vi "溶解氧电极校准.vi"() -> ()   [LabVIEW 2016, in "斯坦道多参数.lvlib"]
uses:
  <vilib>/Utility/miscctls.llb/LVPointTypeDef.ctl
  <vilib>/Analysis/NI_AALBase.lvlib
panel:
  out "第二点校准值":dbl
  out "第一点校准值":dbl
  out "最小值":sgl format="%#.2f"
  out "最大值":sgl format="%#.2f"
  in  "校准模式":enum16{"两点校准", "单点校准"}(ring)=enum."单点校准"
  in  "校准停止":bool
  in  "校准启动":bool
  out "波形图表":sgl(graph) caption="历史曲线"
  out "变异系数":dbl format="%#.6f"
  out "standard deviation":dbl caption="标准差" format="%#.2f"
  out "mean":dbl caption="均值" format="%#.2f"
  out "测量读值":dbl
  out "偏移值补偿":dbl
  out "饱和度值":dbl
  out "提示":string
  out "气压补偿值":dbl
  out "盐度补偿值":dbl
  out "电极斜率":dbl
  out "电极零点":dbl
  # "溶解氧电极设定"
  # "%"
  # "%"
  # "%"
  # "mg/L"
  # "ppt"
  # "hPa"
  # "mg/L"
  # "请选择校准模式:"
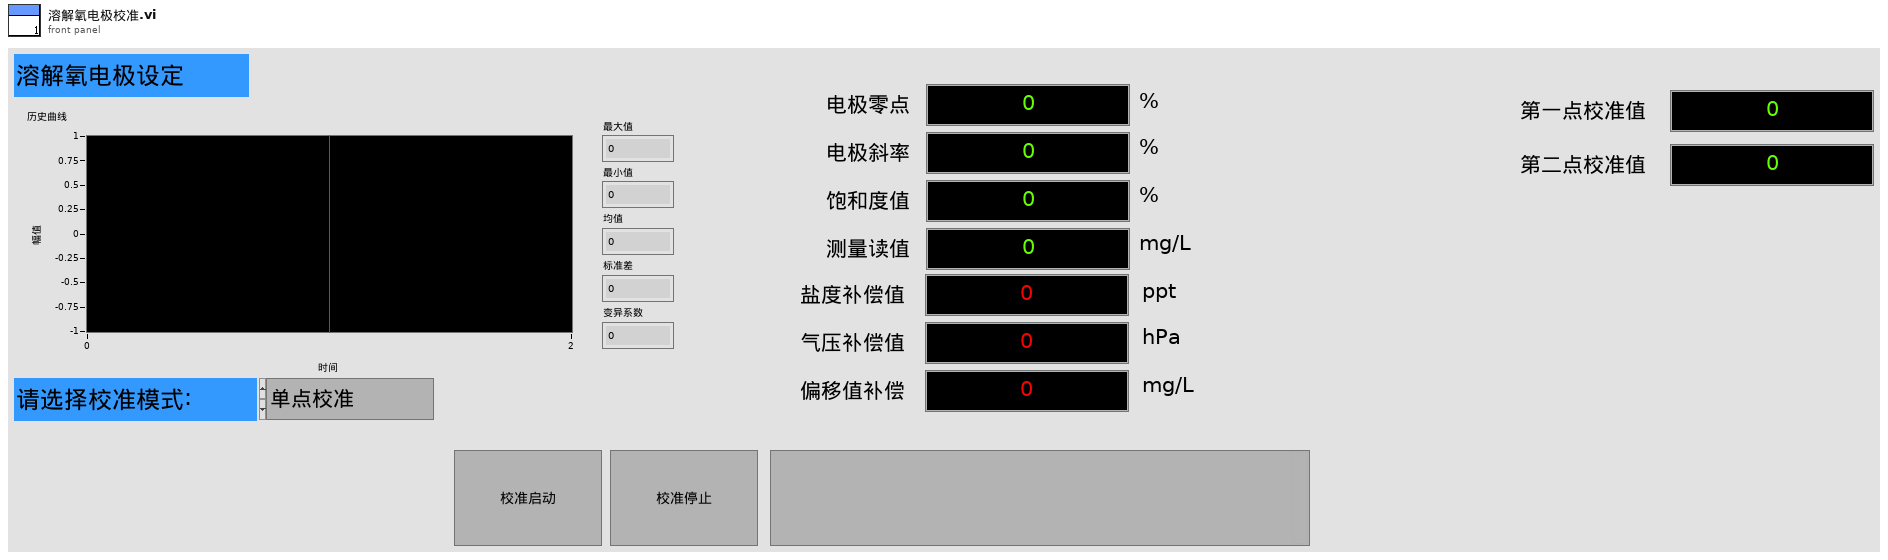
[diagram p1: front panel]
types:
  T1 = typedef "斯坦道多参数.lvlib/校准步骤.ctl" = enum16{"待机", "放置第一点标液", "第一点校准启动", "第一点校准写入", "第一点校准失败", "放置第二点标液", "第二点校准启动", "第二点校准写入", "第二点校准失败", "放置第三点标液", "第三点校准启动", "第三点校准写入", "第三点校准失败", "校准结果写入", "校准结束"}
  T2 = typedef "LVPointTypeDef.ctl" = cluster{"Horizontal":i16, "Vertical":i16}
  T3 = cluster{"电极状态标志":u16, "电极型号标志":u16, "溶解氧测量值":sgl, "温度测量值":sgl, "溶解氧饱和度值":sgl, "盐度补偿值":sgl, "大气压补偿值":sgl, "溶解氧偏移修正值":sgl, "温度偏移修正值":sgl, "手动温度补偿值":sgl, "溶解氧电极零点":sgl, "溶解氧电极斜率":sgl, "第1点标准值记录":sgl, "第1点信号值记录":sgl, "第1点温度值记录":sgl, "第2点标准值记录":sgl, "第2点信号值记录":sgl, "第2点温度值记录":sgl, "命令滤波设定":u16, "温度模式":enum16{"ATC", "MTC"}, "生产批次":u16, "电极序号":u16, "串口地址":u16, "串口波特率":enum16{"9600", "19200", "115200"}, "串口校验位":enum16{"NONE", "ODD", "EVEN"}, "串口停止位":enum16{"1bit", "2bit"}, "第一点标准值":sgl, "第二点标准值":sgl}
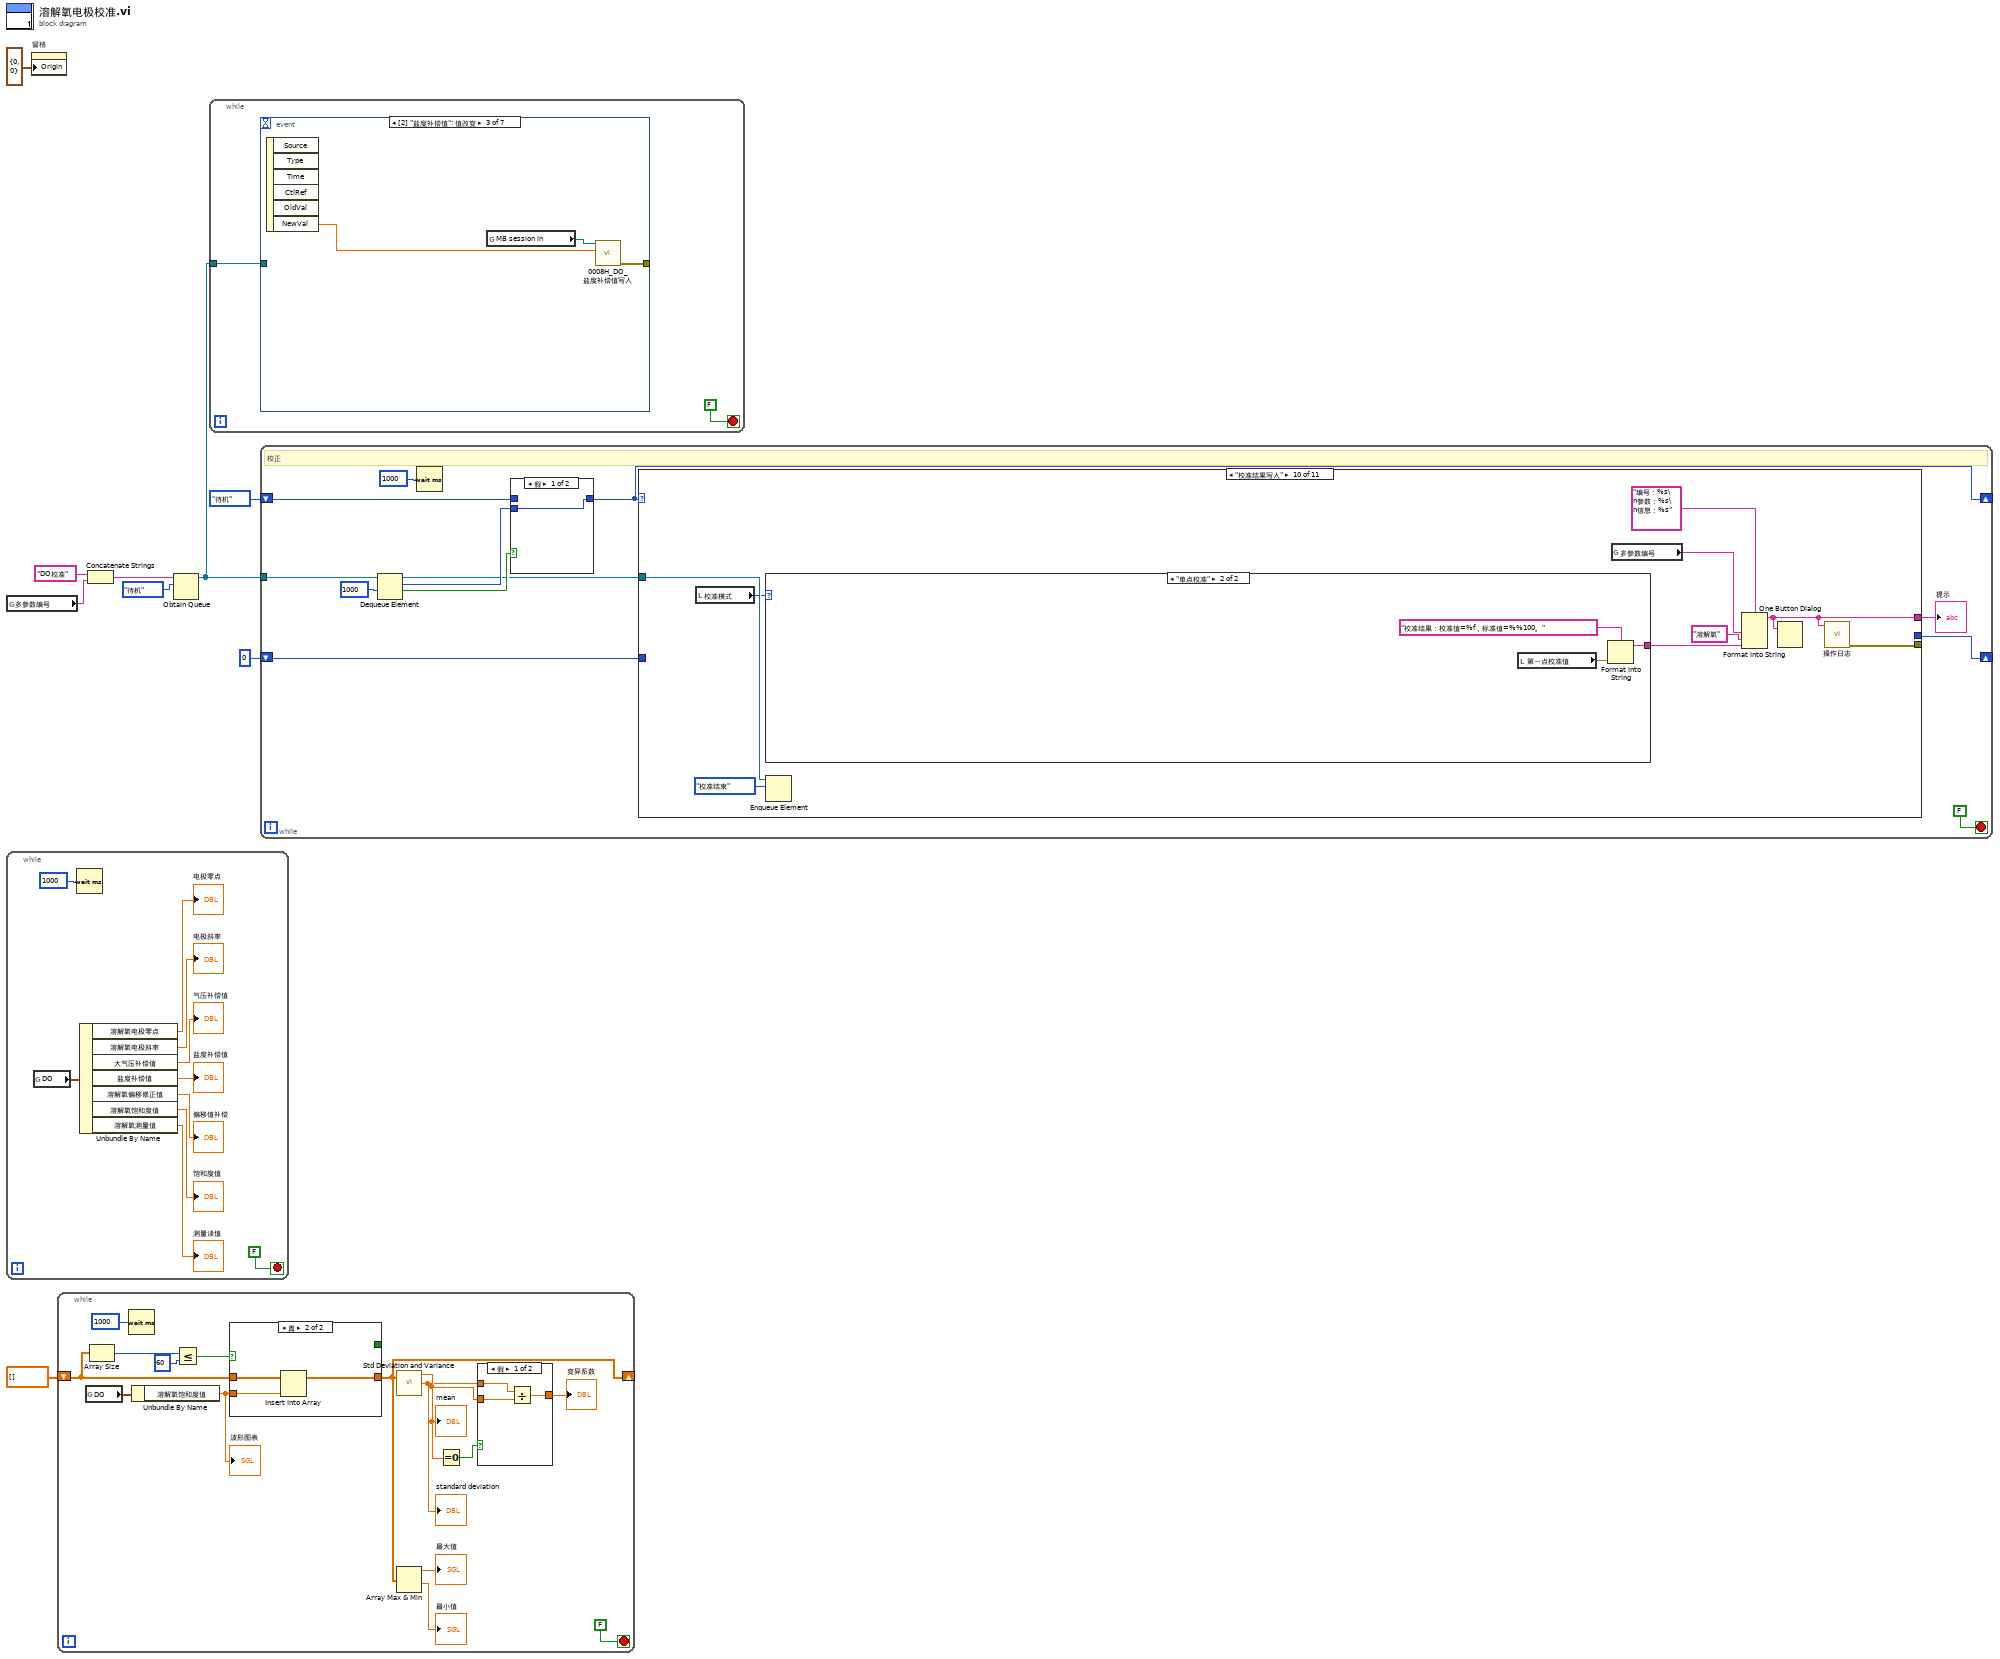
[diagram p0: block diagram]
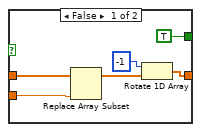
[diagram p3: hidden frame]
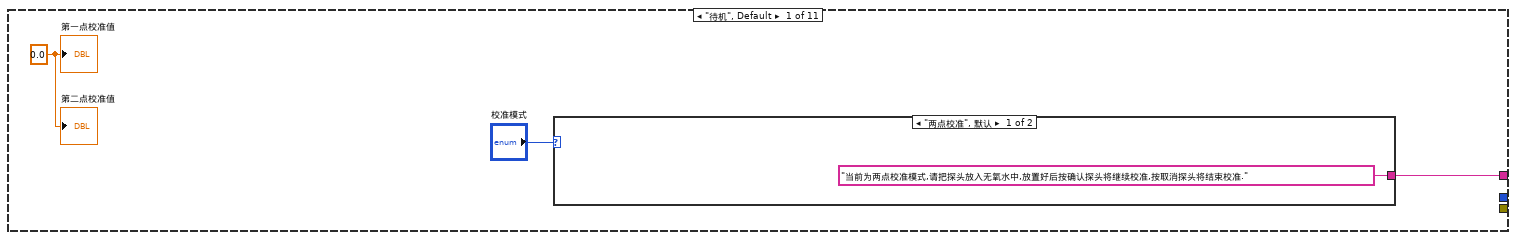
[diagram p5: hidden frame]
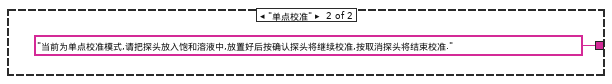
[diagram p6: hidden frame]
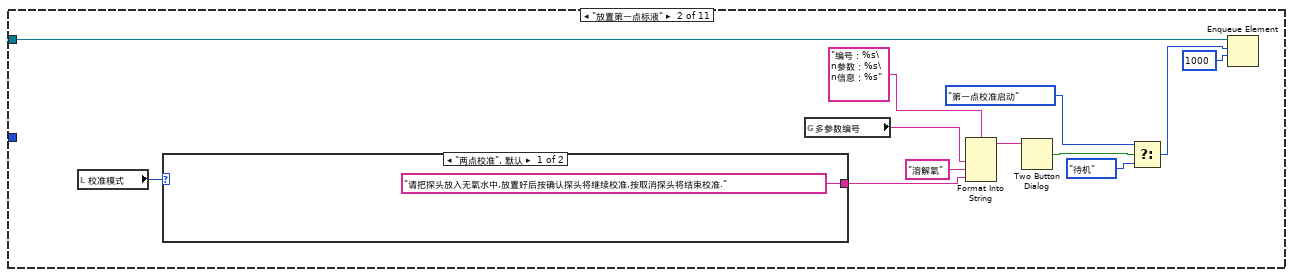
[diagram p7: hidden frame]
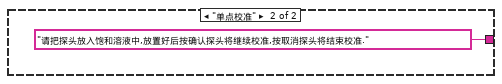
[diagram p8: hidden frame]
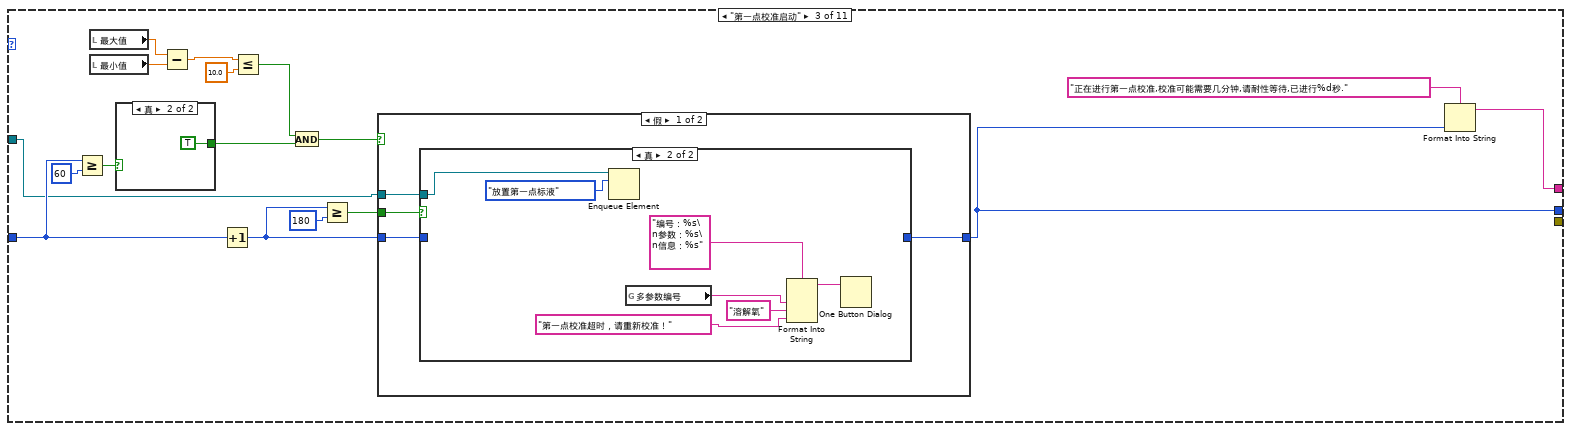
[diagram p9: hidden frame]
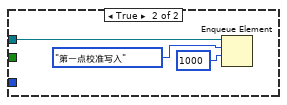
[diagram p11: hidden frame]
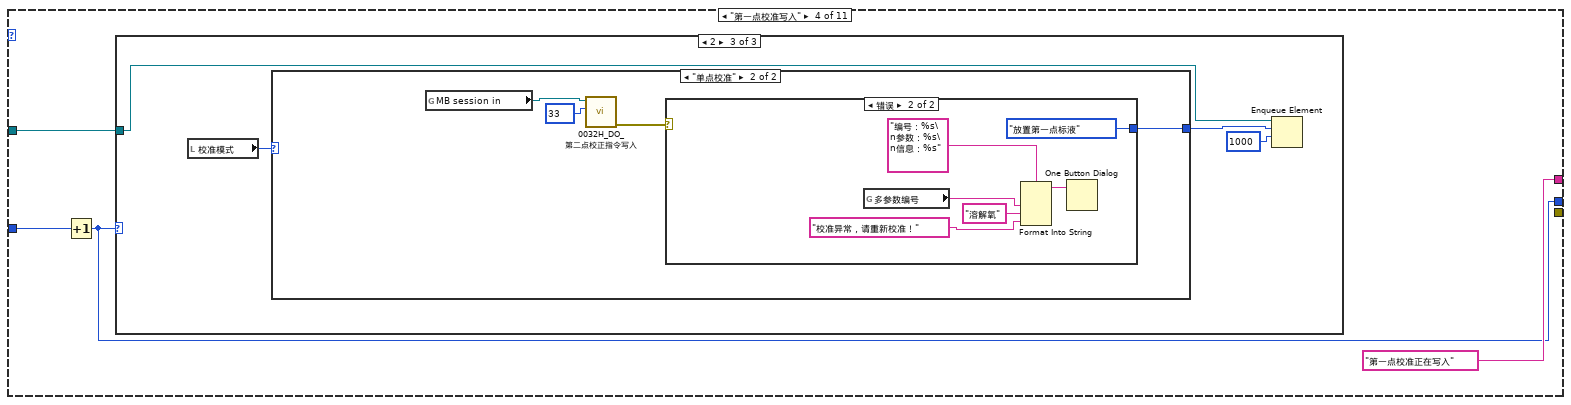
[diagram p13: hidden frame]
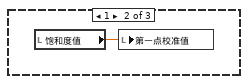
[diagram p15: hidden frame]
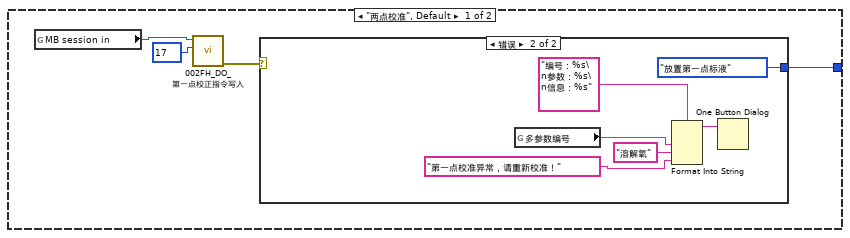
[diagram p16: hidden frame]
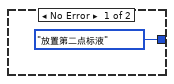
[diagram p17: hidden frame]
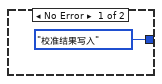
[diagram p18: hidden frame]
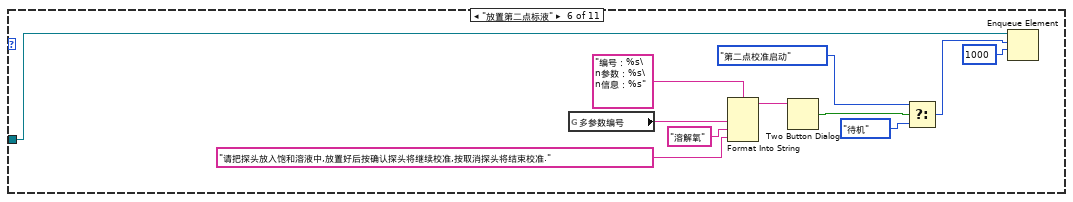
[diagram p20: hidden frame]
diagram:
  n1 = global read "多参数全局变量.vi" "多参数编号"() -> (w1:string)
  n2 = while {
    stop <- FALSE stop-if-true
    n3 = global read "国弘过程全局变量.vi" "DO"() -> (w17:T3)
    n4 = Wait (ms)(milliseconds to wait=u32 1000 ("等待时间（毫秒）")) -> ()  [unwired: 1 out]
    n5 = Unbundle By Name(w17) -> ("溶解氧电极零点"=→"电极零点":sgl, "溶解氧电极斜率"=→"电极斜率":sgl, "大气压补偿值"=→"气压补偿值":sgl, "盐度补偿值"=→"盐度补偿值":sgl, "溶解氧偏移修正值"=→"偏移值补偿":sgl, "溶解氧饱和度值"=→"饱和度值":sgl, "溶解氧测量值"=→"测量读值":sgl)
  }
  n6 = property on="窗格" class="Pane"("Origin"=T2 {"Horizontal"=0, "Vertical"=0} ("原点")) -> ()  [unwired: 2 in, 2 out]
  n7 = while {
    shift-right: [w23] -> _
    shift-left: sgl[] [] -> [w30]
    stop <- FALSE stop-if-true
    n8 = global read "国弘过程全局变量.vi" "DO"() -> (w26:T3)
    n9 = Array Size(array=w30) -> (size(s)=w32:i32)
    n10 = Wait (ms)(milliseconds to wait=u32 1000 ("等待时间（毫秒）")) -> ()  [unwired: 1 out]
    n11 = Unbundle By Name(w26) -> ("溶解氧饱和度值"=w20:sgl)
    "波形图表" <- w20
    n12 = Less Or Equal?(x=w32, y=60) -> (x <= y?=w31:bool)
    n13 = case shown="真" w31 {
      tunnel: w30 -> [w43 w46]
      tunnel: w20 -> [w41 w45]
      tunnel: [w39 w44] -> w23
      tunnel: [TRUE _] -> _
      frame False {
        n14 = Replace Array Subset(array=w43, new element=w41) -> (w42:sgl[])  [unwired: 1 in]
        n15 = Rotate 1D Array(1:w42, 2:-1 ("n")) -> (0:w39:sgl[])
      }
      frame True {
        n16 = Insert Into Array(array=w46, new element=w45) -> (w44:sgl[])  [unwired: 1 in]
      }
    }
    n17 = call <vilib>:"Std Deviation and Variance.vi"("X"=w23) -> ("mean"=w25:dbl, "standard deviation"=w24:dbl)  [unwired: 1 in, 1 out]
    "mean" <- w25
    "standard deviation" <- w24
    n18 = Array Max & Min(array=w23) -> (max value=→"最大值":sgl, min value=→"最小值":sgl)  [unwired: 2 out]
    n19 = Equal To 0?(x=w25) -> (x = 0?=w29:bool)
    n20 = case shown="假" w29 {
      tunnel: w24 -> [w37 _]
      tunnel: [w36 _] -> w28
      tunnel: w25 -> [w35 _]
      frame False {
        n21 = Divide(x=w37, y=w35) -> (x/y=w36:dbl)
      }
      frame True {
      }
    }
    "变异系数" <- w28
  }
  n22 = Concatenate Strings("DO校准" ("名称（未命名）"), w1) -> (w2:string)
  n23 = Obtain Queue(name (unnamed)=w2, element data type=校准步骤."待机" ("枚举")) -> (queue out=w3:refnum<queue>)  [unwired: 3 in, 2 out]
  n24 = while {
    tunnel: w3 -> [w47]
    stop <- FALSE stop-if-true
    n25 = event shown="[2] \"盐度补偿值\": 值改变" {
      selector: _ -> [_ _ _ _ _ _ _]
      dyn-events: _ -> [_ _ _ _ _ _ _]
      timeout: _ -> [_ _ _ _ _ _ _]
      tunnel: [_ _ w54 w57 w60 _ _] -> _
      tunnel: w47 -> [_ _ _ _ _ w62 w64]
      event Timeout {
        n26 = event-data() -> ()  [unwired: 1 in, 3 out]
      }
      event "盐度补偿值", "气压补偿值", "偏移值补偿": Mouse Down {
        n27 = event-data() -> ("CtlRef"=w50:refnum<vi>)  [unwired: 1 in, 7 out]
        n28 = property class="DigNum (严格)"(reference=w50) -> (reference out=w49:refnum<vi>, "Value"=w51:dbl)  [unwired: 1 in, 1 out]
        n29 = call "数字键盘.vi"("OldNumber"=w51) -> ("NewNumber"=w52:dbl)  [unwired: 1 in]
        n30 = property class="DigNum (严格)"(reference=w49, "Val(Sgnl)"=w52) -> ()  [unwired: 1 in, 2 out]
      }
      event "盐度补偿值": Value Change {
        n31 = event-data() -> ("NewVal"=w55:dbl)  [unwired: 1 in, 5 out]
        n32 = global read "多参数全局变量.vi" "MB session in"() -> (w53:refnum<class "MB_Master.lvclass">)
        n33 = call "0008H_DO_盐度补偿值写入.vi"("数值"=w55, "MB session in"=w53) -> ("error out"=w54:errorcluster)  [unwired: 8 in, 1 out]
      }
      event "气压补偿值": Value Change {
        n34 = event-data() -> ("NewVal"=w58:dbl)  [unwired: 1 in, 5 out]
        n35 = global read "多参数全局变量.vi" "MB session in"() -> (w56:refnum<class "MB_Master.lvclass">)
        n36 = call "000AH_DO_大气压补偿值写入.vi"("数值"=w58, "MB session in"=w56) -> ("error out"=w57:errorcluster)  [unwired: 8 in, 1 out]
      }
      event "偏移值补偿": Value Change {
        n37 = event-data() -> ("NewVal"=w61:dbl)  [unwired: 1 in, 5 out]
        n38 = global read "多参数全局变量.vi" "MB session in"() -> (w59:refnum<class "MB_Master.lvclass">)
        n39 = call "000CH_DO_DO偏移修正值写入.vi"("数值"=w61, "MB session in"=w59) -> ("error out"=w60:errorcluster)  [unwired: 8 in, 1 out]
      }
      event "校准启动": Value Change {
        n40 = event-data() -> ()  [unwired: 1 in, 6 out]
        n41 = Enqueue Element(queue=w62, element=校准步骤."放置第一点标液" ("元素")) -> ()  [unwired: 2 in, 3 out]
      }
      event "校准停止": Value Change {
        n42 = event-data() -> ()  [unwired: 1 in, 6 out]
        n43 = Flush Queue(queue=w64) -> (queue out=w65:refnum<queue>)  [unwired: 1 in, 2 out]
        n44 = Enqueue Element(queue=w65, element=校准步骤."待机" ("元素"), timeout in ms (-1)=1000 ("超时毫秒(-1)")) -> ()  [unwired: 1 in, 3 out]
      }
    }
  }
  n45 = while "While循环" {
    shift-right: [w69] -> _
    shift-left: 校准步骤."待机" ("枚举") -> [w70]
    shift-right: [w76] -> _
    shift-left: 0 -> [w77]
    tunnel: w3 -> [w71]
    stop <- FALSE stop-if-true
    # "校正"
    n46 = Dequeue Element(queue=w71, timeout in ms (-1)=1000 ("超时毫秒(-1)")) -> (queue out=w68:refnum<queue>, element=w72:T1, timed out?=w73:bool)  [unwired: 1 in, 1 out]
    n47 = Wait (ms)(milliseconds to wait=u32 1000 ("等待时间（毫秒）")) -> ()  [unwired: 1 out]
    n48 = case shown="假" w73 {
      tunnel: w72 -> [w80 _]
      tunnel: [w80 w81] -> w69
      tunnel: w70 -> [_ w81]
      frame False {
      }
      frame True {
      }
    }
    n49 = case shown="\"校准结果写入\"" w69 {
      tunnel: [w84 _ w105 "第一点校准正在写入" ("提示") _ _ w177 "第二点校准正在写入" ("提示") _ w227 w255] -> w75
      tunnel: w77 -> [_ _ w109 w136 _ _ w179 w211 _ _ _]
      tunnel: [_ _ w108 w135 _ _ w178 w210 _ _ _] -> w76
      tunnel: w68 -> [_ w93 w107 w134 _ w170 w180 w209 _ w234 _]
      tunnel: [_ _ _ _ _ _ _ _ _ w232 _] -> _
      frame "待机", Default {
        w82 = 0.0 ("第一点校准值")
        n50 = case shown="\"两点校准\", 默认" "校准模式" {
          tunnel: ["当前为两点校准模式,请把探头放入无氧水中,放置好后按确认探头将继续校准,按取消探头将结束校准." ("消息") "当前为单点校准模式,请把探头放入饱和溶液中,放置好后按确认探头将继续校准,按取消探头将结束校准." ("消息")] -> w84
          frame "两点校准", Default {
          }
          frame "单点校准" {
          }
        }
        "第一点校准值" <- w82
        "第二点校准值" <- w82
      }
      frame "放置第一点标液" {
        n51 = local read "校准模式"() -> (w92:enum16{"两点校准", "单点校准"})
        n52 = case shown="\"两点校准\", 默认" w92 {
          tunnel: ["请把探头放入无氧水中,放置好后按确认探头将继续校准,按取消探头将结束校准." ("消息") "请把探头放入饱和溶液中,放置好后按确认探头将继续校准,按取消探头将结束校准." ("消息")] -> w87
          frame "两点校准", Default {
          }
          frame "单点校准" {
          }
        }
        n53 = global read "多参数全局变量.vi" "多参数编号"() -> (w90:string)
        n54 = Format Into String(format string="编号：%s\n参数：%s\n信息：%s" ("格式字符串"), w90, "溶解氧" ("输入 2"), w87) -> (resulting string=w88:string)  [unwired: 2 in, 1 out]
        n55 = Two Button Dialog(message=w88) -> (T button?=w97:bool)  [unwired: 2 in]
        n56 = Select(t=校准步骤."第一点校准启动" ("元素"), s=w97, f=校准步骤."待机" ("元素")) -> (s? t:f=w94:T1)
        n57 = Enqueue Element(queue=w93, element=w94, timeout in ms (-1)=1000 ("超时毫秒(-1)")) -> ()  [unwired: 1 in, 3 out]
      }
      frame "第一点校准启动" {
        n58 = Greater Or Equal?(x=w109, y=60) -> (x >= y?=w116:bool)
        n59 = local read "最大值"() -> (w113:sgl)
        n60 = local read "最小值"() -> (w112:sgl)
        n61 = case shown="真" w116 {
          tunnel: [_ TRUE] -> w104
          frame False {
          }
          frame True {
          }
        }
        n62 = Subtract(x=w113, y=w112) -> (x-y=w114:sgl)
        n63 = Increment(x=w109) -> (x+1=w106:i32)
        n64 = Less Or Equal?(x=w114, y=10.0) -> (x <= y?=w103:bool)
        n65 = And(x=w103, y=w104) -> (x .and. y?=w102:bool)
        n66 = Greater Or Equal?(x=w106, y=180) -> (x >= y?=w110:bool)
        n67 = case shown="假" w102 {
          tunnel: w107 -> [w120 w132]
          tunnel: w110 -> [w121 _]
          tunnel: w106 -> [w119 _]
          tunnel: [w118 _] -> w108
          frame False {
            n68 = case shown="真" w121 {
              tunnel: w120 -> [_ w129]
              tunnel: w119 -> [w122 _]
              tunnel: [w122 _] -> w118
              frame False {
              }
              frame True {
                n69 = Enqueue Element(queue=w129, element=校准步骤."放置第一点标液" ("元素")) -> ()  [unwired: 2 in, 3 out]
                n70 = global read "多参数全局变量.vi" "多参数编号"() -> (w126:string)
                n71 = Format Into String(format string="编号：%s\n参数：%s\n信息：%s" ("格式字符串"), w126, "溶解氧" ("输入 2"), "第一点校准超时，请重新校准！" ("error source (\" \")")) -> (resulting string=w124:string)  [unwired: 2 in, 1 out]
                n72 = One Button Dialog(message=w124) -> ()  [unwired: 1 in, 1 out]
              }
            }
          }
          frame True {
            n73 = Enqueue Element(queue=w132, element=校准步骤."第一点校准写入" ("元素"), timeout in ms (-1)=1000 ("超时毫秒(-1)")) -> ()  [unwired: 1 in, 3 out]
          }
        }
        n74 = Format Into String(format string="正在进行第一点校准,校准可能需要几分钟,请耐性等待,已进行%d秒." ("格式字符串"), w108) -> (resulting string=w105:string)  [unwired: 2 in, 1 out]
      }
      frame "第一点校准写入" {
        n75 = Increment(x=w136) -> (x+1=w135:i32)
        n76 = case shown="2" w135 {
          tunnel: w134 -> [_ _ w140]
          frame 0, Default {
          }
          frame 1 {
            n77 = local read "饱和度值"() -> (w138:dbl)
            n78 = local write "第一点校准值"(w138) -> ()
          }
          frame 2 {
            n79 = local read "校准模式"() -> (w142:enum16{"两点校准", "单点校准"})
            n80 = case shown="\"单点校准\"" w142 {
              tunnel: [w143 w154] -> w139
              frame "两点校准", Default {
                n81 = global read "多参数全局变量.vi" "MB session in"() -> (w144:refnum<class "MB_Master.lvclass">)
                n82 = call "002FH_DO_第一点校正指令写入.vi"("数值"=u16 17, "MB session in"=w144) -> ("error out"=w145:errorcluster)  [unwired: 8 in, 1 out]
                n83 = case shown="错误" w145 {
                  tunnel: [校准步骤."放置第二点标液" ("元素") 校准步骤."放置第一点标液" ("元素")] -> w143
                  frame No Error {
                  }
                  frame Error {
                    n84 = global read "多参数全局变量.vi" "多参数编号"() -> (w151:string)
                    n85 = Format Into String(format string="编号：%s\n参数：%s\n信息：%s" ("格式字符串"), w151, "溶解氧" ("输入 2"), "第一点校准异常，请重新校准！" ("error source (\" \")")) -> (resulting string=w149:string)  [unwired: 2 in, 1 out]
                    n86 = One Button Dialog(message=w149) -> ()  [unwired: 1 in, 1 out]
                  }
                }
              }
              frame "单点校准" {
                n87 = global read "多参数全局变量.vi" "MB session in"() -> (w156:refnum<class "MB_Master.lvclass">)
                n88 = call "0032H_DO_第二点校正指令写入.vi"("数值"=u16 33, "MB session in"=w156) -> ("error out"=w155:errorcluster)  [unwired: 8 in, 1 out]
                n89 = case shown="错误" w155 {
                  tunnel: [校准步骤."校准结果写入" ("元素") 校准步骤."放置第一点标液" ("元素")] -> w154
                  frame No Error {
                  }
                  frame Error {
                    n90 = global read "多参数全局变量.vi" "多参数编号"() -> (w162:string)
                    n91 = Format Into String(format string="编号：%s\n参数：%s\n信息：%s" ("格式字符串"), w162, "溶解氧" ("输入 2"), "校准异常，请重新校准！" ("error source (\" \")")) -> (resulting string=w161:string)  [unwired: 2 in, 1 out]
                    n92 = One Button Dialog(message=w161) -> ()  [unwired: 1 in, 1 out]
                  }
                }
              }
            }
            n93 = Enqueue Element(queue=w140, element=w139, timeout in ms (-1)=1000 ("超时毫秒(-1)")) -> ()  [unwired: 1 in, 3 out]
          }
        }
      }
      frame "第一点校准失败" {
      }
      frame "放置第二点标液" {
        n94 = global read "多参数全局变量.vi" "多参数编号"() -> (w168:string)
        n95 = Format Into String(format string="编号：%s\n参数：%s\n信息：%s" ("格式字符串"), w168, "溶解氧" ("输入 2"), "请把探头放入饱和溶液中,放置好后按确认探头将继续校准,按取消探头将结束校准." ("消息")) -> (resulting string=w165:string)  [unwired: 2 in, 1 out]
        n96 = Two Button Dialog(message=w165) -> (T button?=w174:bool)  [unwired: 2 in]
        n97 = Select(t=校准步骤."第二点校准启动" ("元素"), s=w174, f=校准步骤."待机" ("元素")) -> (s? t:f=w171:T1)
        n98 = Enqueue Element(queue=w170, element=w171, timeout in ms (-1)=1000 ("超时毫秒(-1)")) -> ()  [unwired: 1 in, 3 out]
      }
      frame "第二点校准启动" {
        n99 = Greater Or Equal?(x=w179, y=60) -> (x >= y?=w191:bool)
        n100 = local read "最大值"() -> (w188:sgl)
        n101 = local read "最小值"() -> (w187:sgl)
        n102 = case shown="真" w191 {
          tunnel: [_ TRUE] -> w184
          frame False {
          }
          frame True {
          }
        }
        n103 = Subtract(x=w188, y=w187) -> (x-y=w189:sgl)
        n104 = Increment(x=w179) -> (x+1=w185:i32)
        n105 = Less Or Equal?(x=w189, y=10.0) -> (x <= y?=w183:bool)
        n106 = And(x=w183, y=w184) -> (x .and. y?=w182:bool)
        n107 = Greater Or Equal?(x=w185, y=180) -> (x >= y?=w186:bool)
        n108 = case shown="假" w182 {
          tunnel: w180 -> [w195 w207]
          tunnel: w186 -> [w196 _]
          tunnel: w185 -> [w194 _]
          tunnel: [w193 _] -> w178
          frame False {
            n109 = case shown="真" w196 {
              tunnel: w195 -> [_ w204]
              tunnel: w194 -> [w197 _]
              tunnel: [w197 _] -> w193
              frame False {
              }
              frame True {
                n110 = Enqueue Element(queue=w204, element=校准步骤."放置第二点标液" ("元素")) -> ()  [unwired: 2 in, 3 out]
                n111 = global read "多参数全局变量.vi" "多参数编号"() -> (w201:string)
                n112 = Format Into String(format string="编号：%s\n参数：%s\n信息：%s" ("格式字符串"), w201, "溶解氧" ("输入 2"), "第二点校准超时，请重新校准！" ("error source (\" \")")) -> (resulting string=w199:string)  [unwired: 2 in, 1 out]
                n113 = One Button Dialog(message=w199) -> ()  [unwired: 1 in, 1 out]
              }
            }
          }
          frame True {
            n114 = Enqueue Element(queue=w207, element=校准步骤."第二点校准写入" ("元素"), timeout in ms (-1)=1000 ("超时毫秒(-1)")) -> ()  [unwired: 1 in, 3 out]
          }
        }
        n115 = Format Into String(format string="正在进行第二点校准,校准可能需要几分钟,请耐性等待,已进行%d秒." ("格式字符串"), w178) -> (resulting string=w177:string)  [unwired: 2 in, 1 out]
      }
      frame "第二点校准写入" {
        n116 = Increment(x=w211) -> (x+1=w210:i32)
        n117 = case shown="2" w210 {
          tunnel: w209 -> [_ _ w214]
          frame 0, Default {
            (unwired) 校准步骤."第二点校准写入" ("枚举")
          }
          frame 1 {
            n118 = local read "饱和度值"() -> (w213:dbl)
            n119 = local write "第二点校准值"(w213) -> ()
          }
          frame 2 {
            n120 = global read "多参数全局变量.vi" "MB session in"() -> (w218:refnum<class "MB_Master.lvclass">)
            n121 = call "0032H_DO_第二点校正指令写入.vi"("数值"=u16 33, "MB session in"=w218) -> ("error out"=w215:errorcluster)  [unwired: 8 in, 1 out]
            n122 = case shown="错误" w215 {
              tunnel: [校准步骤."校准结果写入" ("元素") 校准步骤."放置第二点标液" ("元素")] -> w216
              frame No Error {
              }
              frame Error {
                n123 = global read "多参数全局变量.vi" "多参数编号"() -> (w224:string)
                n124 = Format Into String(format string="编号：%s\n参数：%s\n信息：%s" ("格式字符串"), w224, "溶解氧" ("输入 2"), "第二点校准异常，请重新校准！" ("error source (\" \")")) -> (resulting string=w222:string)  [unwired: 2 in, 1 out]
                n125 = One Button Dialog(message=w222) -> ()  [unwired: 1 in, 1 out]
              }
            }
            n126 = Enqueue Element(queue=w214, element=w216, timeout in ms (-1)=1000 ("超时毫秒(-1)")) -> ()  [unwired: 1 in, 3 out]
          }
        }
      }
      frame "第二点校准失败" {
      }
      frame "校准结果写入" {
        n127 = local read "校准模式"() -> (w233:enum16{"两点校准", "单点校准"})
        n128 = case shown="\"单点校准\"" w233 {
          tunnel: [w236 w254] -> w228
          frame "两点校准", Default {
            n129 = global read "国弘过程全局变量.vi" "DO"() -> (w238:T3)
            n130 = Unbundle By Name(w238) -> ("电极状态标志"=w237:u16)
            n131 = case shown="2" w237 {
              selector: w237 -> [w240 _ w249]
              tunnel: [w239 w246 w248] -> w236
              frame 0, Default {
                n132 = case shown="2" w240 {
                  tunnel: ["校正未正常启动，请重新校正" "第一点校准通过" "第二点校准通过"] -> w239
                  frame 0, Default {
                  }
                  frame 1 {
                  }
                  frame 2 {
                  }
                }
              }
              frame 2 {
                n133 = local read "第一点校准值"() -> (w247:dbl)
                n134 = local read "第二点校准值"() -> (w244:dbl)
                n135 = Format Into String(format string="校准结果：第一点校准值=%f，第一点标准值=%%0,第二点校准值=%f，第二点标准值=%%100." ("提示"), w247, w244) -> (resulting string=w246:string)  [unwired: 2 in, 1 out]
              }
              frame 3, 4 {
                n136 = case shown="4" w249 {
                  tunnel: ["校正失败，电极零点超出范围" "校正失败，电极斜率超出范围"] -> w248
                  frame 3, Default {
                  }
                  frame 4 {
                  }
                }
              }
            }
          }
          frame "单点校准" {
            n137 = local read "第一点校准值"() -> (w253:dbl)
            n138 = Format Into String(format string="校准结果：校准值=%f，标准值=%%100。" ("提示"), w253) -> (resulting string=w254:string)  [unwired: 2 in, 1 out]
          }
        }
        n139 = Enqueue Element(queue=w234, element=校准步骤."校准结束" ("元素")) -> ()  [unwired: 2 in, 3 out]
        n140 = global read "多参数全局变量.vi" "多参数编号"() -> (w230:string)
        n141 = Format Into String(format string="编号：%s\n参数：%s\n信息：%s" ("格式字符串"), w230, "溶解氧" ("输入 2"), w228) -> (resulting string=w227:string)  [unwired: 2 in, 1 out]
        n142 = One Button Dialog(message=w227) -> ()  [unwired: 1 in, 1 out]
        n143 = call "操作日志.vi"("日志信息"=w227) -> ("error out"=w232:errorcluster)  [unwired: 10 in]
      }
      frame "校准结束" {
        n144 = local read "提示"() -> (w255:string)
      }
    }
    "提示" <- w75
  }
